vi "AcquireImage.vi"(8 "error in (no error)":errorcluster, 10 "image in":T2, 11 "session in":T1) -> (0 "error out":errorcluster, 1 "timestamp":timestamp, 2 "image out":T2, 3 "session out":T1)   [LabVIEW 2017, in "IrAcquisition.lvlib"]
uses:
  <vilib>/addons/InsightCM/Devices/Shared/Ir/IrAcquisition/IrAcquisition.lvlib
  <vilib>/vision/Image Controls.llb/IMAQ Image.ctl
  <vilib>/userdefined/High Color/IMAQdx.ctl
  <vilib>/vision/driver/NI_Vision_Acquisition_Software.lvlib
  <vilib>/vision/driver/IMAQdx.llb/IMAQdx Buffer Number Mode.ctl
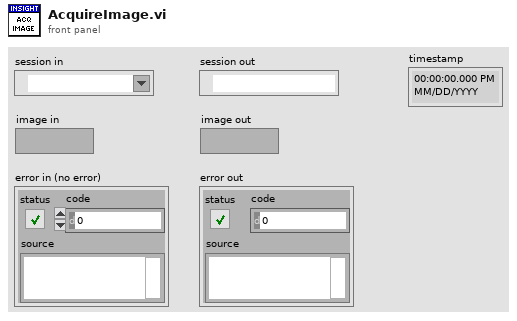
[diagram p1: front panel]
types:
  T1 = typedef "IMAQdx.ctl" = refnum<k21>
  T2 = typedef "IMAQ Image.ctl" = refnum<image>
  T3 = typedef "NI_Vision_Acquisition_Software.lvlib/IMAQdx Buffer Number Mode.ctl" = enum32{"Next", "Last", "Buffer Number", "Every", "Last New"}
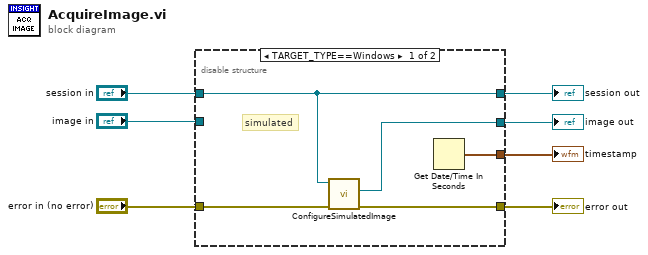
[diagram p0: block diagram]
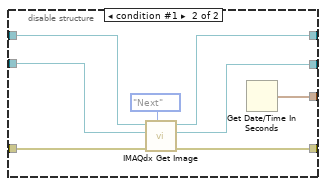
[diagram p2: hidden frame]
diagram:
  n1 = disable-structure shown="TARGET_TYPE==Windows" {
    disable-tunnel: "image in" -> [_ w20]
    disable-tunnel: [w9 w19] -> w2
    disable-tunnel: [w8 w18] -> w6
    disable-tunnel: [w10 w17] -> w5
    disable-tunnel: "session in" -> [w8 w16]
    disable-tunnel: "error in (no error)" -> [w11 w15]
    disable-tunnel: [w12 w14] -> w1
    frame condition #0 (active) {
      # "simulated"
      n2 = call <vilib>:"ConfigureSimulatedImage.vi"("error in (no error)"=w11, "Camera SN"=w8) -> ("error out"=w10:errorcluster, "image"=w9:T2)  [unwired: 8 in]
      n3 = Get Date/Time In Seconds() -> (seconds since 1Jan1904=w12:timestamp)
    }
    frame condition #1 {
      n4 = call <vilib>:"IMAQdx Get Image.vi"("Buffer Number Mode (Next)"=IMAQdx_Buffer_Number_Mode."Next", "error in"=w15, "Image In"=w20, "Session In"=w16) -> ("error out"=w17:errorcluster, "Image Out"=w19:T2, "Session Out"=w18:T1)  [unwired: 1 in, 4 out]
      n5 = Get Date/Time In Seconds() -> (seconds since 1Jan1904=w14:timestamp)
    }
  }
  "image out" <- w2
  "session out" <- w6
  "error out" <- w5
  "timestamp" <- w1
